vi "Get Rx Tx resources.vi"(0 "resources":T3[](array[typedef]), 5 "direction":T4, 11 "error in (no error)":errorcluster) -> (4 "RX Resources":T1[](array[typedef]), 6 "TX Resources":T1[](array[typedef]), 15 "error out":errorcluster)   [LabVIEW 2019]
uses:
  TypeDefs/Direction.ctl
  TypeDefs/Resources.ctl
  <vilib>/userdefined/High Color/nirio_resource_hc.ctl
  TypeDefs/Baseband Resources.ctl
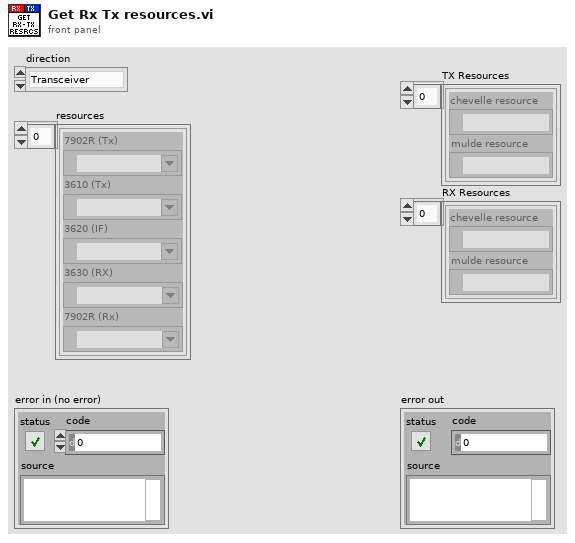
[diagram p1: front panel]
types:
  T1 = typedef "Baseband Resources.ctl" = cluster{"chevelle resource":T2, "mulde resource":refnum<visa-resource-name>}
  T2 = typedef "nirio_resource_hc.ctl" = tag
  T3 = typedef "Resources.ctl" = cluster{"7902R (Tx)":T2, "3610 (Tx)":refnum<visa-resource-name>, "3620 (IF)":T2, "3630 (RX)":refnum<visa-resource-name>, "7902R (Rx)":T2}
  T4 = typedef "Direction.ctl" = enum16{"Transceiver", "Receiver", "Transmitter"}
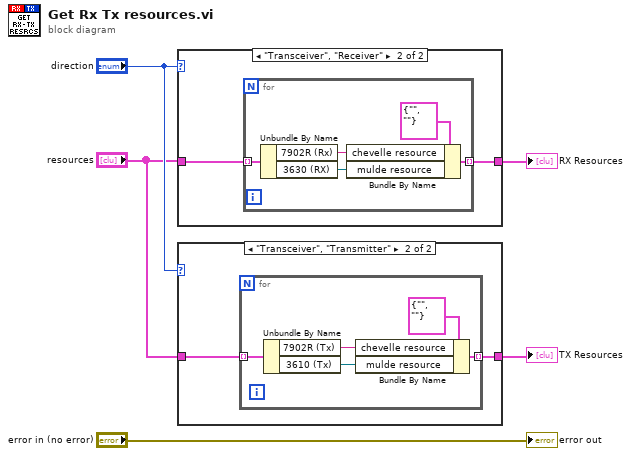
[diagram p0: block diagram]
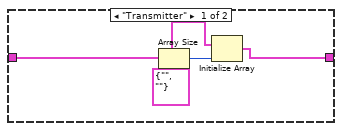
[diagram p2: hidden frame]
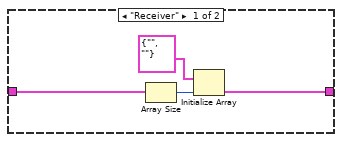
[diagram p3: hidden frame]
diagram:
  n1 = case shown="\"Transceiver\", \"Receiver\"" "direction" {
    tunnel: "resources" -> [w9 w11]
    tunnel: [w6 w10] -> w2
    frame "Transmitter" {
      n2 = Array Size(array=w9) -> (size(s)=w8:i32)
      n3 = Initialize Array(T1 {"chevelle resource"="", "mulde resource"=""} ("tx resources"), w8) -> (w6:T1[])
    }
    frame "Transceiver", "Receiver" {
      n4 = for {
        tunnel: w11 -> [w16] mode=indexing
        tunnel: [w13] -> w10 mode=indexing
        n5 = Unbundle By Name(w16) -> ("7902R (Rx)"=w15:T2, "3630 (RX)"=w14:refnum<visa-resource-name>)
        n6 = Bundle By Name(cluster=T1 {"chevelle resource"="", "mulde resource"=""} ("tx resources"), "chevelle resource"=w15, "mulde resource"=w14) -> (w13:T1)
      }
    }
  }
  "RX Resources" <- w2
  n7 = case shown="\"Transceiver\", \"Transmitter\"" "direction" {
    tunnel: "resources" -> [w20 w22]
    tunnel: [w17 w21] -> w3
    frame "Receiver" {
      n8 = Array Size(array=w20) -> (size(s)=w19:i32)
      n9 = Initialize Array(T1 {"chevelle resource"="", "mulde resource"=""} ("tx resources"), w19) -> (w17:T1[])
    }
    frame "Transceiver", "Transmitter" {
      n10 = for {
        tunnel: w22 -> [w27] mode=indexing
        tunnel: [w24] -> w21 mode=indexing
        n11 = Unbundle By Name(w27) -> ("7902R (Tx)"=w26:T2, "3610 (Tx)"=w25:refnum<visa-resource-name>)
        n12 = Bundle By Name(cluster=T1 {"chevelle resource"="", "mulde resource"=""} ("tx resources"), "chevelle resource"=w26, "mulde resource"=w25) -> (w24:T1)
      }
    }
  }
  "TX Resources" <- w3
  "error out" <- "error in (no error)"
